vi "ReferenceMove Core.vi"(8 "error in (no error)":errorcluster, 10 "AxisNumber":u8, 11 "CS++SimMotor in":refnum<class "CS++SimMotor.lvclass">) -> (0 "error out":errorcluster, 3 "CS++SimMotor out":refnum<class "CS++SimMotor.lvclass">)   [LabVIEW 2015, in "CS++SimMotor.lvlib" / "CS++SimMotor.lvclass"]
doc: "Starts a movement to the reference switch of this axis. Once the motor reaches the reference switch it should slowly move down from the switch and stop. Afterwards the internal step counter is set to zero. \n\nThe main purpose of this function is to calibrate the motor."
uses:
  CS++SimMotor.lvclass
  CS++SimMotor.lvclass/CS++SimMotor.ctl
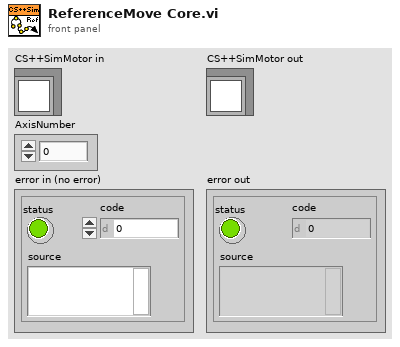
[diagram p1: front panel]
types:
  T1 = enum16{"RelativeMovement", "AbsoluteMovement", "Stop", "ReferenceMovement"}
  T2 = cluster{"AxisNumber":u8, dbl, "Enum":enum16{"RelativeMovement", "AbsoluteMovement", "Stop", "ReferenceMovement"}}
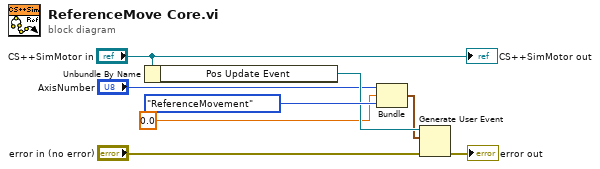
[diagram p0: block diagram]
diagram:
  n1 = Unbundle By Name("CS++SimMotor in") -> ("Pos Update Event"=w7:refnum<user-event>)
  n2 = Bundle("AxisNumber"="AxisNumber", 0.0, "Enum"=T1."ReferenceMovement") -> (w6:T2)  [unwired: 1 in]
  n3 = Generate User Event(user event=w7, event data cluster=w6, error in="error in (no error)") -> (error out=→"error out":errorcluster)  [unwired: 1 in, 1 out]
  "CS++SimMotor out" <- "CS++SimMotor in"
